vi "Status Relay Condition.vi"(0 "VISA resource name":refnum<visa-resource-name>, 11 "error in (no error)":errorcluster) -> (4 "VISA resource name out":refnum<visa-resource-name>, 8 "Relay Status":T1, 15 "error out":errorcluster)   [LabVIEW 2012, in "Lake Shore Cryotronics 218.lvlib"]
doc: "This VI indicates the status of the 218 relays. Only the model 218S includes the relays."
uses:
  <instrlib>/Lake Shore Cryotronics 218/Lake Shore Cryotronics 218.lvlib
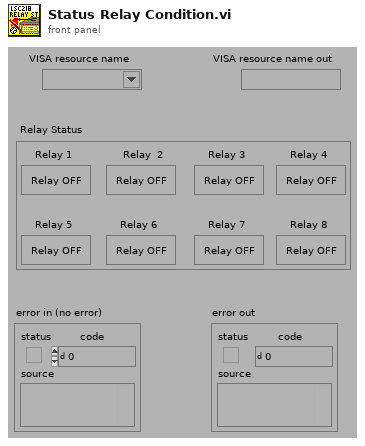
[diagram p1: front panel]
types:
  T1 = cluster{"Relay 1":bool, "Relay  2":bool, "Relay 3":bool, "Relay 4":bool, "Relay 5":bool, "Relay 6":bool, "Relay 7":bool, "Relay 8":bool}
  T2 = cluster{"Boolean array[0]":bool, "Boolean array[1]":bool, "Boolean array[2]":bool, "Boolean array[3]":bool, "Boolean array[4]":bool, "Boolean array[5]":bool, "Boolean array[6]":bool, "Boolean array[7]":bool}
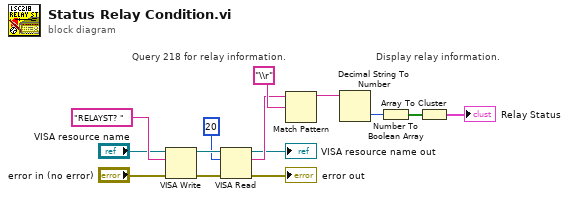
[diagram p0: block diagram]
diagram:
  # "Query 218 for relay information."
  # "Display relay information."
  n1 = VISA Write(VISA resource name="VISA resource name", write buffer="RELAYST? ", error in (no error)="error in (no error)") -> (VISA resource name out=w14:refnum<visa-resource-name>, error out=w13:errorcluster)  [unwired: 1 out]
  n2 = VISA Read(VISA resource name=w14, byte count=20, error in (no error)=w13) -> (VISA resource name out=→"VISA resource name out":refnum<visa-resource-name>, read buffer=w11:string, error out=→"error out":errorcluster)  [unwired: 1 out]
  n3 = Match Pattern(string=w11, regular expression="\\r") -> (before substring=w6:string)  [unwired: 1 in, 3 out]
  n4 = Decimal String To Number(string=w6) -> (number=w8:i32)  [unwired: 2 in, 1 out]
  n5 = Number To Boolean Array(number=w8) -> (Boolean array=w9:bool[])
  n6 = Array To Cluster(array=w9) -> (cluster=→"Relay Status":T2)
